vi "Write Variables for Control.vi"(4 "Motors Enable":bool[](array[boolean])=[FALSE, FALSE, FALSE], 6 "Tension Control":bool=TRUE, 8 "Start, End Point":bool[](array[boolean]), 9 "Target Stop":bool, 10 "Encoder Initialize":bool, 11 "Trajectory":i32(slide) scale=0.0..2.0) -> ()   [LabVIEW 2021]
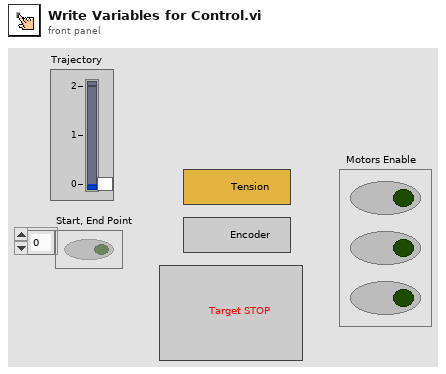
[diagram p1: front panel]
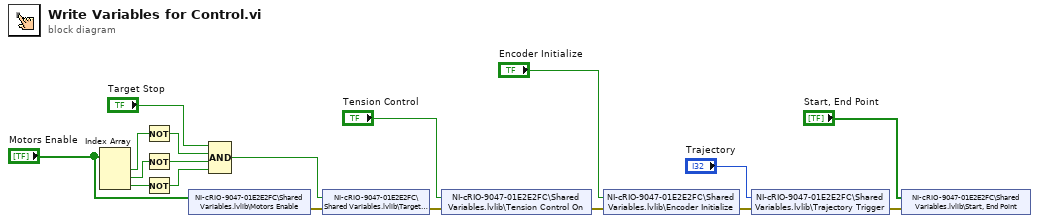
[diagram p0: block diagram]
diagram:
  n1 = Index Array(array="Motors Enable") -> (element #1=w8:bool, element #2=w5:bool, element #3=w4:bool)  [unwired: 3 in]
  n2 = Not(x=w8) -> (.not. x?=w7:bool)
  n3 = Not(x=w5) -> (.not. x?=w6:bool)
  n4 = Not(x=w4) -> (.not. x?=w3:bool)
  n5 = shared-variable "NI-cRIO-9047-01E2E2FC\\Shared Variables.lvlib\\Motors Enable"("Motors Enable") -> (error out=w13:errorcluster)  [unwired: 1 in]
  n6 = Compound Arithmetic op=AND("Target Stop", w7, w6, w3) -> (w1:bool)
  n7 = shared-variable "NI-cRIO-9047-01E2E2FC\\Shared Variables.lvlib\\Target Stop"(w1, error in=w13) -> (error out=w12:errorcluster)
  n8 = shared-variable "NI-cRIO-9047-01E2E2FC\\Shared Variables.lvlib\\Tension Control On"("Tension Control", error in=w12) -> (error out=w17:errorcluster)
  n9 = shared-variable "NI-cRIO-9047-01E2E2FC\\Shared Variables.lvlib\\Encoder Initialize"("Encoder Initialize", error in=w17) -> (error out=w18:errorcluster)
  n10 = shared-variable "NI-cRIO-9047-01E2E2FC\\Shared Variables.lvlib\\Trajectory Trigger"("Trajectory", error in=w18) -> (error out=w10:errorcluster)
  n11 = shared-variable "NI-cRIO-9047-01E2E2FC\\Shared Variables.lvlib\\Start, End Point"("Start, End Point", error in=w10) -> ()  [unwired: 1 out]
